vi "Write Caption Ref.vi"(8 "error in (no error)":errorcluster, 10 "Caption":string, 11 "Power Meter Display in":refnum<class "Power Meter Display.lvclass">) -> (0 "error out":errorcluster, 3 "Power Meter Display out":refnum<class "Power Meter Display.lvclass">)   [LabVIEW 2012]
uses:
  Power Meter Display.lvclass
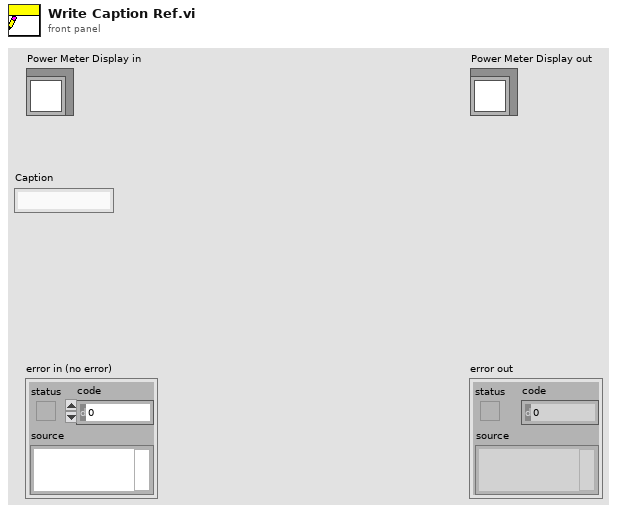
[diagram p1: front panel]
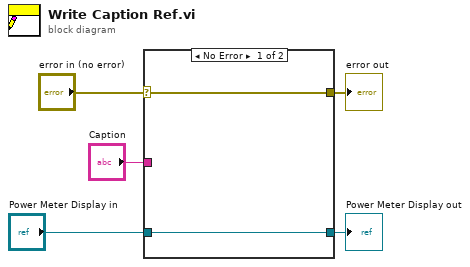
[diagram p0: block diagram]
diagram:
  n1 = case shown="No Error" "error in (no error)" {
    selector: "error in (no error)" -> [w7 w8]
    tunnel: [w7 w8] -> w4
    tunnel: [w6 w9] -> w2
    tunnel: "Power Meter Display in" -> [w6 w9]
    tunnel: "Caption" -> [_ _]
    frame No Error {
    }
    frame Error {
    }
  }
  "error out" <- w4
  "Power Meter Display out" <- w2
